vi "Create Per Hour Between Datetime.vi"(11 "befor N day of Current day":dbl) -> (3 "per Hour Between SQL":string[](array[string]))   [LabVIEW 2021]
uses:
  <userlib>/LabSQL/LabSQL.lvlib
panel:
  out "resulting string":string
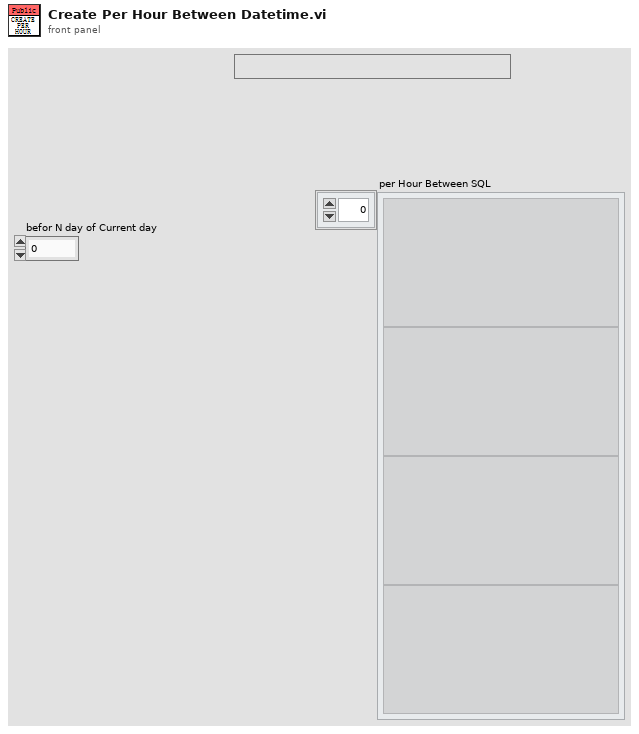
[diagram p1: front panel]
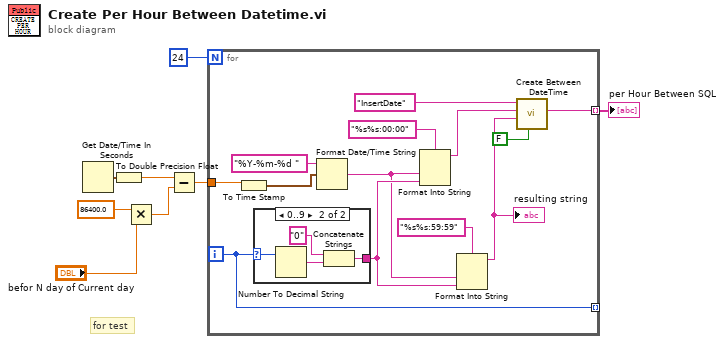
[diagram p0: block diagram]
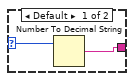
[diagram p2: hidden frame]
diagram:
  # "for test"
  n1 = Get Date/Time In Seconds() -> (seconds since 1Jan1904=w6:timestamp)
  n2 = To Double Precision Float(number=w6) -> (double precision float=w5:dbl)
  n3 = Multiply(x=86400.0, y="befor N day of Current day") -> (x*y=w3:dbl)
  n4 = Subtract(x=w5, y=w3) -> (x-y=w2:dbl)
  n5 = for {
    N: 24 -> [_]
    tunnel: [w20] -> w1 mode=indexing
    tunnel: w2 -> [w11]
    tunnel: [w9] -> _ mode=indexing
    i -> [w9]
    n6 = To Time Stamp(1:w11) -> (0:w10:timestamp)
    n7 = case shown="0..9" w9 {
      selector: w9 -> [w23 w27]
      tunnel: [w22 w24] -> w16
      frame Default {
        n8 = Number To Decimal String(number=w23) -> (decimal integer string=w22:string)  [unwired: 1 in]
      }
      frame 0..9 {
        n9 = Number To Decimal String(number=w27) -> (decimal integer string=w26:string)  [unwired: 1 in]
        n10 = Concatenate Strings("0" ("string"), w26) -> (w24:string)
      }
    }
    n11 = Format Date/Time String(time format string (%c)="%Y-%m-%d ", seconds (now)=w10) -> (date/time string=w15:string)  [unwired: 1 in]
    n12 = Format Into String(format string="%s%s:00:00", w15, w16) -> (resulting string=w14:string)  [unwired: 2 in, 1 out]
    n13 = Format Into String(format string="%s%s:59:59", w15, w16) -> (resulting string=w13:string)  [unwired: 2 in, 1 out]
    "resulting string" <- w13
    n14 = call <userlib>:"Create Between DateTime.vi"("HaveWhere?"=FALSE, "End DateTime"=w13, "Start DateTime"=w14, "Column Name"="InsertDate") -> ("Between DateTime"=w20:string)  [unwired: 7 in]
  }
  "per Hour Between SQL" <- w1
